vi "Kelly.vi"() -> ()   [LabVIEW 2016]
panel:
  in  "Add=+ divide=/ multiply=x subtract=-":string
  in  "Numeric 3":dbl
  in  "Numeric 2":dbl
  out "Numeric":dbl
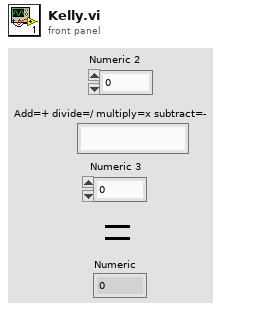
[diagram p1: front panel]
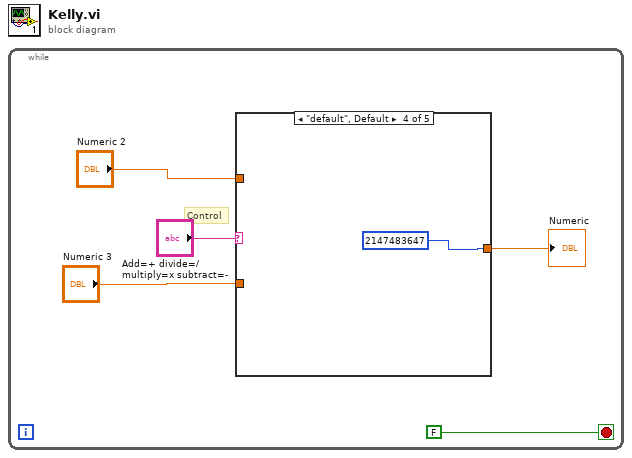
[diagram p0: block diagram]
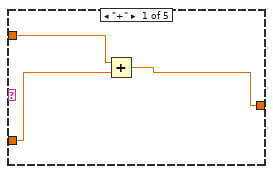
[diagram p2: hidden frame]
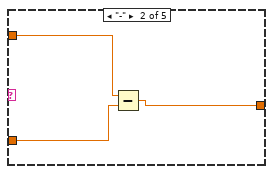
[diagram p3: hidden frame]
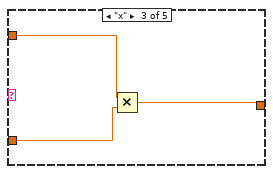
[diagram p4: hidden frame]
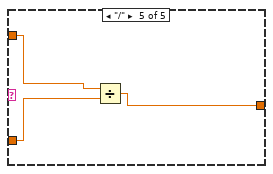
[diagram p5: hidden frame]
diagram:
  n1 = while {
    stop <- FALSE stop-if-true
    # "Control"
    n2 = case shown="\"default\", Default" "Add=+ divide=/ multiply=x subtract=-" {
      tunnel: "Numeric 3" -> [w7 w10 w14 _ w17]
      tunnel: "Numeric 2" -> [w8 w11 w13 _ w18]
      tunnel: [w6 w9 w12 2147483647 w16] -> w2
      frame "+" {
        n3 = Add(x=w8, y=w7) -> (x+y=w6:dbl)
      }
      frame "-" {
        n4 = Subtract(x=w11, y=w10) -> (x-y=w9:dbl)
      }
      frame "x" {
        n5 = Multiply(x=w13, y=w14) -> (x*y=w12:dbl)
      }
      frame "default", Default {
      }
      frame "/" {
        n6 = Divide(x=w18, y=w17) -> (x/y=w16:dbl)
      }
    }
    "Numeric" <- w2
  }
